vi "Core Recieve Message.vi"(7 "Message Priority":T1=enum."Normal", 8 "error in (no error)":errorcluster, 9 "Message":refnum<class "Message.lvclass">, 10 "Actor in":refnum<class "Actor.lvclass">, 11 "Instrument Sequencer in":refnum<class "Instrument Sequencer.lvclass">) -> (0 "error out":errorcluster, 2 "Actor out":refnum<class "Actor.lvclass">, 3 "Instrument Sequencer out":refnum<class "Instrument Sequencer.lvclass">)   [LabVIEW 2020, in "Instrument Handler.lvlib" / "Instrument Sequencer.lvclass"]
doc: "Recieve the dequeued message.\nThe default implementation executes the Message Do method."
uses:
  Instrument Sequencer.lvclass
  PPL/HDH.Actor Framework.Core.Actor.lvlibp/1abvi3w/vi.lib/ActorFramework/Message Enqueuer/Message Priority.ctl
  PPL/HDH.Actor Framework.Core.Actor.lvlibp/1abvi3w/vi.lib/ActorFramework/Message/Message.lvclass
  PPL/HDH.Actor Framework.Core.Actor.lvlibp/1abvi3w/vi.lib/ActorFramework/Actor/Actor.lvclass
  Instrument Owner/Instrument Owner.lvclass
  C:/Current projects/WS/PPL/HDH.Actor Framework.Core.Actor.lvlibp/1abvi3w/vi.lib/ActorFramework/Actor/Actor.lvclass
  Messages/Instrument Msg/Instrument Msg.lvclass
  C:/Current projects/WS/PPL/HDH.Actor Framework.Core.Actor.lvlibp/1abvi3w/vi.lib/ActorFramework/Message/Message.lvclass
  Instrument Sequencer.lvclass/Instrument Sequencer.ctl
  PPL/HDH.Actor Framework.Core.Sequencer.lvlibp/Sequencer/Read Core.vi
  PPL/HDH.Actor Framework.Core.Instrument Driver.lvlibp/Instrument Driver/Instrument Driver.lvclass
  PPL/HDH.Actor Framework.Core.Sequencer.lvlibp/Sequencer Core/Sequencer Core.lvclass
  Instrument Handler.lvlib
  PPL/HDH.Actor Framework.Core.Actor.lvlibp/1abvi3w/vi.lib/ActorFramework/Message Enqueuer/Message Enqueuer.lvclass
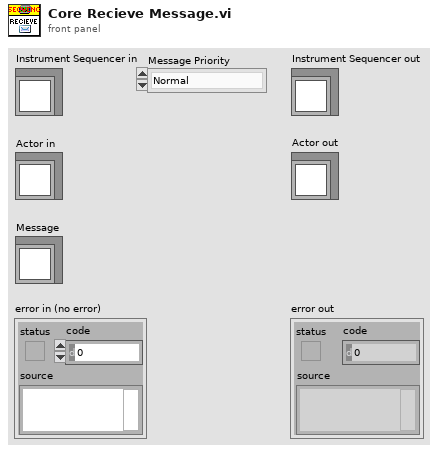
[diagram p1: front panel]
types:
  T1 = typedef "HDH.Actor Framework.Core.Actor.lvlibp/Message Enqueuer.lvclass/Message Priority.ctl" = enum16{"Low", "Normal", "High"}
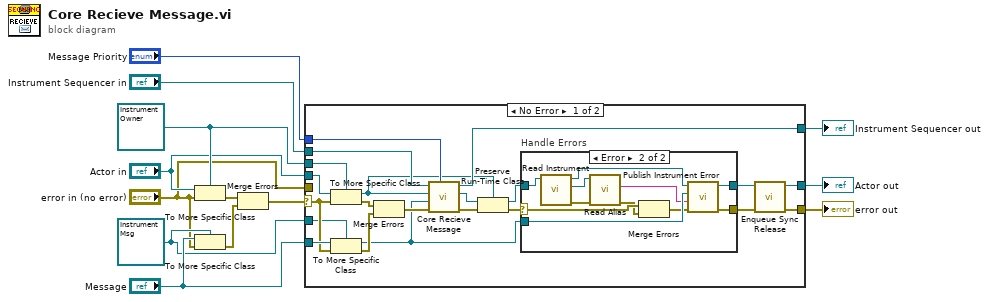
[diagram p0: block diagram]
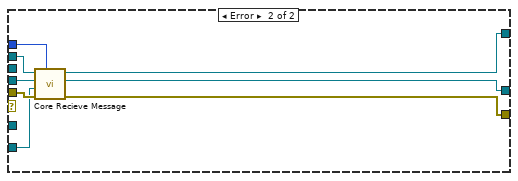
[diagram p3: hidden frame]
diagram:
  w2 = refnum<class "Instrument Msg.lvclass"> refnum ("Instrument Handler.lvlib:Instrument Msg.lvclass")
  w7 = refnum<class "Instrument Owner.lvclass"> refnum ("Instrument Handler.lvlib:Instrument Owner.lvclass")
  n1 = To More Specific Class(target class=w7, reference="Actor in", error in="error in (no error)") -> (error out=w8:errorcluster)  [unwired: 1 out]
  n2 = To More Specific Class(target class=w2, reference="Message", error in="error in (no error)") -> (error out=w4:errorcluster)  [unwired: 1 out]
  n3 = Merge Errors(w8, w4) -> (w5:errorcluster)
  n4 = case shown="No Error" w5 {
    selector: w5 -> [w24 _]
    tunnel: [w28 w48] -> w13
    tunnel: [w31 w49] -> w12
    tunnel: [w34 w52] -> w11
    tunnel: "Message Priority" -> [w33 w50]
    tunnel: "Message" -> [w25 w51]
    tunnel: "Instrument Sequencer in" -> [w32 w53]
    tunnel: w7 -> [w27 _]
    tunnel: "Actor in" -> [w26 w54]
    tunnel: w2 -> [w23 _]
    tunnel: "error in (no error)" -> [_ w55]
    frame No Error {
      n5 = To More Specific Class(target class=w27, reference=w26, error in=w24) -> (specific class reference=w19:refnum<class "Instrument Owner.lvclass">, error out=w22:errorcluster)
      n6 = To More Specific Class(target class=w23, reference=w25, error in=w24) -> (specific class reference=w14:refnum<class "Instrument Msg.lvclass">, error out=w21:errorcluster)
      n7 = Merge Errors(w22, w21) -> (w20:errorcluster)
      n8 = call-parent "Core Recieve Message.vi"("Message Priority"=w33, "error in (no error)"=w20, "Message"=w14, "Actor in"=w19, "Sequencer Core in"=w32) -> ("error out"=w29:errorcluster, "Actor out"=w30:refnum<class "Actor.lvclass">, "Sequencer Core out"=w34:refnum<class "Instrument Sequencer.lvclass">)  [unwired: 4 in]
      n9 = Preserve Run-Time Class(object in=w30, error in=w29, 2:w19) -> (object out=w16:refnum<class "Instrument Owner.lvclass">, error out=w18:errorcluster)
      n10 = case "Handle Errors" shown="Error" w18 {
        selector: w18 -> [w36 w47]
        tunnel: [w36 w46] -> w17
        tunnel: w16 -> [w35 w43]
        tunnel: [w35 w45] -> w15
        tunnel: w14 -> [_ w44]
        frame No Error {
        }
        frame Error {
          n11 = call "Read Instrument.vi"("Instrument Owner in"=w43) -> ("error out"=w40:errorcluster, "Instrument out"=w41:refnum<class "Instrument Driver.lvclass">, "Instrument Owner out"=w42:refnum<class "Instrument Owner.lvclass">)  [unwired: 8 in]
          n12 = call "Read Alias.vi"("error in (no error)"=w40, "Instrument in"=w41) -> ("error out"=w37:errorcluster, "Alias"=w39:string)  [unwired: 7 in, 1 out]
          n13 = Merge Errors(w47, w37) -> (w38:errorcluster)
          n14 = call "Publish Instrument Error.vi"("error in (no error)"=w38, "Instrument String"=w39, "Instrument Msg"=w44, "Actor in"=w42) -> ("error out"=w46:errorcluster, "Actor out"=w45:refnum<class "Instrument Owner.lvclass">)  [unwired: 6 in]
        }
      }
      n15 = call "Enqueue Sync Release.vi"("error in (no error)"=w17, "Instrument Owner in"=w15) -> ("error out"=w28:errorcluster, "Instrument Owner out"=w31:refnum<class "Instrument Owner.lvclass">)  [unwired: 8 in]
    }
    frame Error {
      n16 = call-parent "Core Recieve Message.vi"("Message Priority"=w50, "error in (no error)"=w55, "Message"=w51, "Actor in"=w54, "Sequencer Core in"=w53) -> ("error out"=w48:errorcluster, "Actor out"=w49:refnum<class "Actor.lvclass">, "Sequencer Core out"=w52:refnum<class "Instrument Sequencer.lvclass">)  [unwired: 4 in]
    }
  }
  "error out" <- w13
  "Instrument Sequencer out" <- w11
  "Actor out" <- w12
